vi "SetSerializableData.vi"(7 "BlueSerializer in":refnum<class "BlueSerializer.lvclass">, 8 "error in (no error)":errorcluster, 10 "Data In":T1={"StructuredData"=variant(string ""), "ClassOps (child, parent)"=[]}, 11 "BlueSerializable in":refnum<class "BlueSerializable.lvclass">) -> (0 "error out":errorcluster, 2 "Data Out":T1={"StructuredData"=variant(string ""), "ClassOps (child, parent)"=[]}, 3 "BlueSerializable out":refnum<class "BlueSerializable.lvclass">, 5 "BlueSerializer out":refnum<class "BlueSerializer.lvclass">)   [LabVIEW 2020, in "BlueSerialization.lvlib" / "BlueSerializable.lvclass"]
doc: "Dynamic Dispatch setter to set SerializableData for all inheritance levels of a <b>BlueSerializable</b> class. This and all overrides should ONLY be consumed by a child of <b>SerializerBase</b>"
uses:
  BlueSerializable.lvclass
  BlueSerializer/Support/SetSerializableDataCluster.ctl
  BlueSerializer/Support/SetSerializableDataClusterIterable.ctl
  BlueSerializer/Support/SetSerializableDataClusterLayer.ctl
  BlueSerializer/BlueSerializableVersion.ctl
  BlueSerializer/Support/SetSerializableDataObject.ctl
  BlueSerializer/BlueSerializer.lvclass
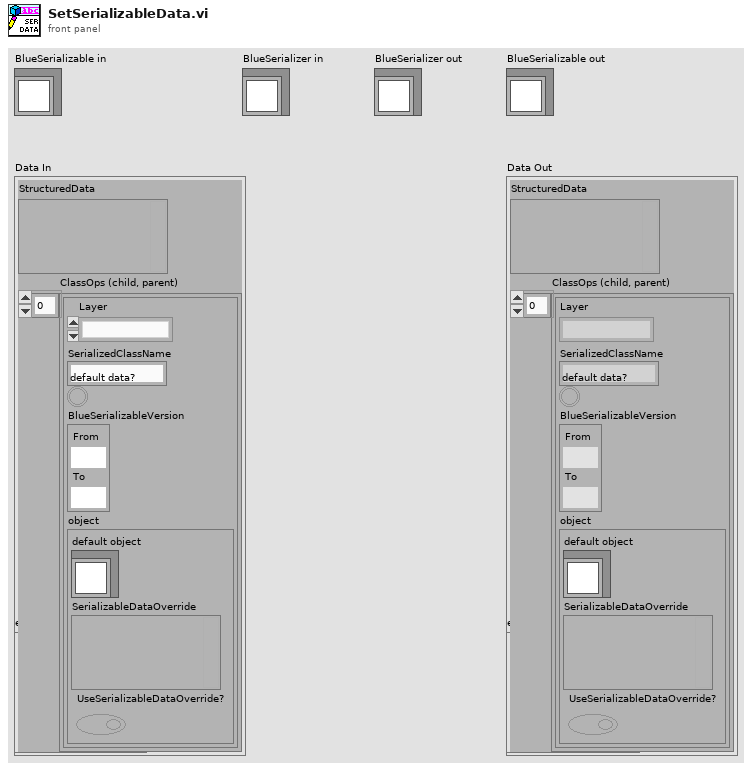
[diagram p1: front panel]
types:
  T1 = typedef "BlueSerialization.lvlib/BlueSerializer.lvclass/SetSerializableDataCluster.ctl" = cluster{"StructuredData":variant, "ClassOps (child, parent)":T2[]}
  T2 = typedef "BlueSerialization.lvlib/BlueSerializer.lvclass/SetSerializableDataClusterIterable.ctl" = cluster{"Layer":T3, "SerializedClassName":string, "default data?":bool, "BlueSerializableVersion":T4, "object":T5}
  T3 = typedef "BlueSerialization.lvlib/BlueSerializer.lvclass/SetSerializableDataClusterLayer.ctl" = enum16{"new class layer", "dropped class layer", "agreed class layer"}
  T4 = typedef "BlueSerialization.lvlib/BlueSerializer.lvclass/BlueSerializableVersion.ctl" = cluster{"From":u16, "To":u16}
  T5 = typedef "BlueSerialization.lvlib/BlueSerializer.lvclass/SetSerializableDataObject.ctl" = cluster{"default object":refnum<class "BlueSerializable.lvclass">, "SerializableDataOverride":variant, "UseSerializableDataOverride?":bool}
  T6 = typedef "BlueSerialization.lvlib/BlueSerializable.lvclass/SerializableData.ctl" = cluster{"LibVersion":u8}
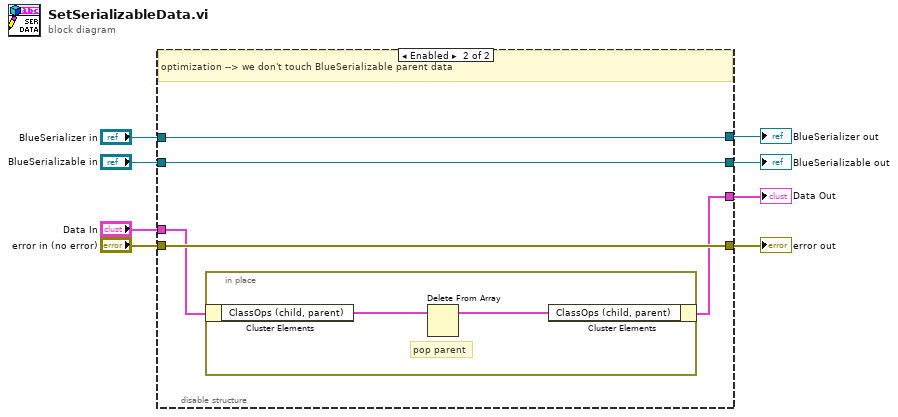
[diagram p0: block diagram]
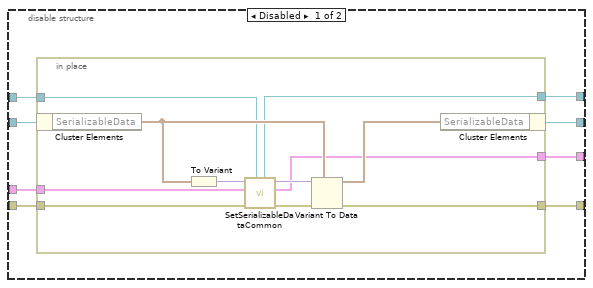
[diagram p2: hidden frame]
diagram:
  n1 = disable-structure shown="Enabled" {
    disable-tunnel: "BlueSerializable in" -> [w16 w31]
    disable-tunnel: "Data In" -> [w15 w29]
    disable-tunnel: "error in (no error)" -> [w14 w30]
    disable-tunnel: [w13 w31] -> w5
    disable-tunnel: [w12 w28] -> w4
    disable-tunnel: [w11 w30] -> w3
    disable-tunnel: "BlueSerializer in" -> [w10 w32]
    disable-tunnel: [w9 w32] -> w1
    frame Disabled {
      n2 = in-place {
        in-place-border: w14 -> [w21]
        in-place-border: [w26] -> w11
        in-place-border: w15 -> [w24]
        in-place-border: [w19] -> w12
        in-place-border: w10 -> [w18]
        in-place-border: [w17] -> w9
        n3 = in-place-cluster #1(w16) -> ("SerializableData"=w23:T6)
        n4 = To Variant(anything=w23) -> (Variant=w22:variant)
        n5 = call "SetSerializableDataCommon.vi"("BlueSerializer in"=w18, "error in (no error)"=w21, "Data In"=w24, "SerializableData"=w22) -> ("error out"=w25:errorcluster, "Data Out"=w19:T1, "SerializableData"=w20:variant, "BlueSerializer out"=w17:refnum<class "BlueSerializer.lvclass">)  [unwired: 4 in]
        n6 = Variant To Data(error in=w25, type=w23, Variant=w20) -> (data=w27:T6, error out=w26:errorcluster)
        n7 = in-place-cluster #1("SerializableData"=w27) -> (w13:refnum<class "BlueSerializable.lvclass">)
      }
    }
    frame Enabled {
      # "optimization --> we don't touch BlueSerializable parent data"
      n8 = in-place {
        # "pop parent"
        n9 = in-place-cluster #2(w29) -> ("ClassOps (child, parent)"=w34:T2[])
        n10 = Delete From Array(array=w34) -> (array with subset deleted=w33:T2[])  [unwired: 2 in, 1 out]
        n11 = in-place-cluster #2("ClassOps (child, parent)"=w33) -> (w28:T1)
      }
    }
  }
  "error out" <- w3
  "BlueSerializable out" <- w5
  "Data Out" <- w4
  "BlueSerializer out" <- w1
